vi "Get End Point.vi"(8 "error in (no error)":errorcluster, 10 "End":enum16{"Source", "Target"}(ring), 11 "FSM.Edge in":refnum<class "FSM.Edge.lvclass">) -> (0 "error out":errorcluster, 2 "point":cluster{"x":i16, "y":i16}, 3 "FSM.Edge out":refnum<class "FSM.Edge.lvclass">)   [LabVIEW 2015, in "FSM.Edge.lvclass"]
uses:
  FSM.Edge.lvclass
  FSM.Edge.lvclass/FSM.Edge.ctl
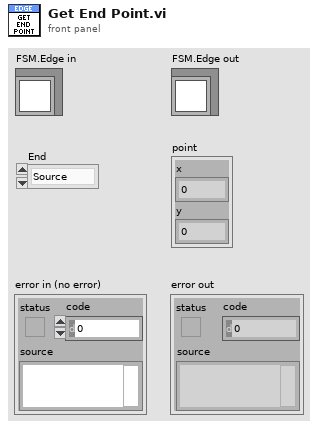
[diagram p1: front panel]
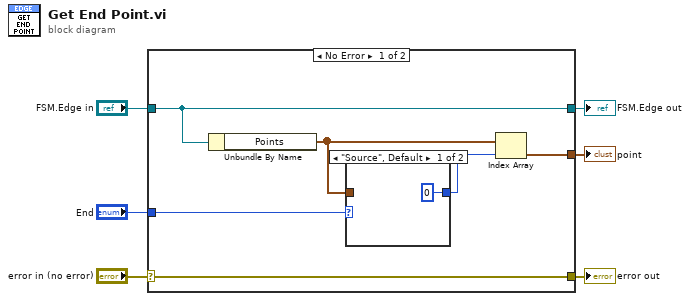
[diagram p0: block diagram]
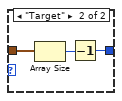
[diagram p2: hidden frame]
diagram:
  n1 = case shown="No Error" "error in (no error)" {
    selector: "error in (no error)" -> [w12 w18]
    tunnel: [w12 w18] -> w5
    tunnel: [w11 w17] -> w3
    tunnel: "FSM.Edge in" -> [w11 w17]
    tunnel: "End" -> [w10 _]
    tunnel: [w7 _] -> w1
    frame No Error {
      n2 = Unbundle By Name(w11) -> ("Points"=w9:cluster{"x":i16, "y":i16}[])
      n3 = case shown="\"Source\", Default" w10 {
        tunnel: w9 -> [_ w16]
        tunnel: [0 w14] -> w8
        frame "Source", Default {
        }
        frame "Target" {
          n4 = Array Size(array=w16) -> (size(s)=w15:i32)
          n5 = Decrement(x=w15) -> (x-1=w14:i32)
        }
      }
      n6 = Index Array(array=w9, index=w8) -> (element=w7:cluster{"x":i16, "y":i16})
    }
    frame Error {
    }
  }
  "error out" <- w5
  "FSM.Edge out" <- w3
  "point" <- w1
